vi "log.vi"(8 "error in (no error)":errorcluster, 10 "log_entry":T1 {"datetime" format="%<%x %.3X>T"}, 11 "console.provider in":refnum<class "console.provider.lvclass">) -> (0 "error out":errorcluster, 3 "console.provider out":refnum<class "console.provider.lvclass">)   [LabVIEW 2021, in "console.provider.lvclass"]
uses:
  console.provider.lvclass
  Z:/Projects/DIT/lv-default-repo/source/system.logging.provider/system.logging.provider.lvclass
  system.logging/log_entry.ctl
  system.logging/severity.ctl
  system.logging.provider.lvclass/system.logging.provider.ctl
  console.provider.lvclass/console.provider.ctl
  system.logging.provider.lvclass
  system.logging/system.logging.lvclass
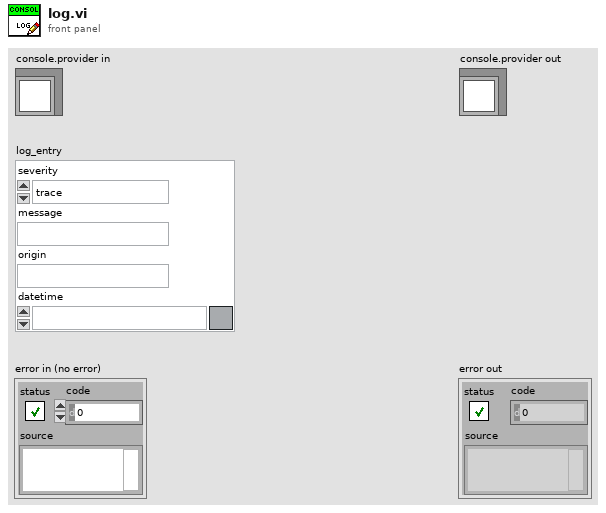
[diagram p1: front panel]
types:
  T1 = typedef "system.logging.lvclass/log_entry.ctl" = cluster{"severity":T2, "message":string, "origin":string, "datetime":timestamp}
  T2 = typedef "system.logging.lvclass/severity.ctl" = enum8{"trace", "debug", "info", "warning", "error"}
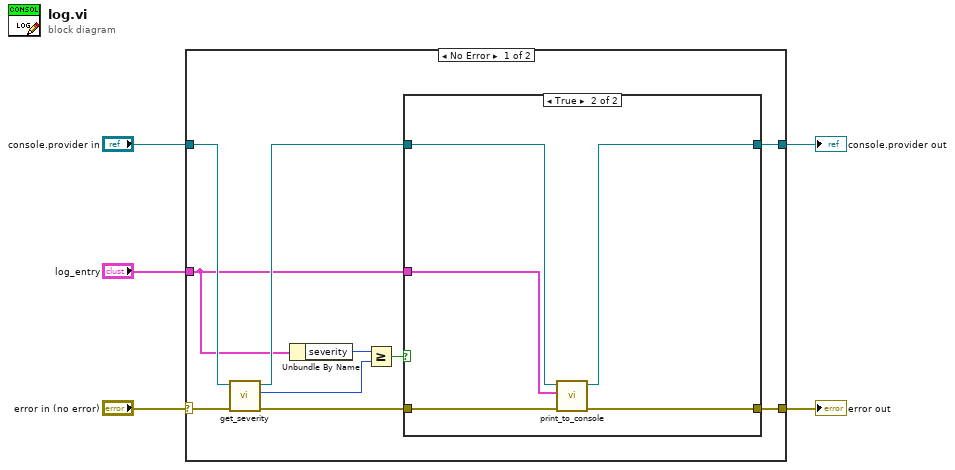
[diagram p0: block diagram]
diagram:
  n1 = case shown="No Error" "error in (no error)" {
    selector: "error in (no error)" -> [w15 w24]
    tunnel: [w8 w24] -> w1
    tunnel: [w7 w23] -> w4
    tunnel: "console.provider in" -> [w14 w23]
    tunnel: "log_entry" -> [w6 _]
    frame No Error {
      n2 = call "get_severity.vi"("error in (no error)"=w15, "system.logging.provider in"=w14) -> ("error out"=w10:errorcluster, "severity"=w12:T2, "system.logging.provider out"=w9:refnum<class "console.provider.lvclass">)  [unwired: 7 in]
      n3 = Unbundle By Name(w6) -> ("severity"=w13:T2)
      n4 = Greater Or Equal?(x=w13, y=w12) -> (x >= y?=w11:bool)
      n5 = case shown="True" w11 {
        tunnel: w10 -> [w17 w22]
        tunnel: w9 -> [w16 w21]
        tunnel: [w17 w18] -> w8
        tunnel: [w16 w20] -> w7
        tunnel: w6 -> [_ w19]
        frame False {
          # "Discard, entry"
        }
        frame True {
          n6 = call "print_to_console.vi"("error in (no error)"=w22, "log"=w19, "console.provider in"=w21) -> ("error out"=w18:errorcluster, "console.provider out"=w20:refnum<class "console.provider.lvclass">)  [unwired: 7 in]
        }
      }
    }
    frame Error {
    }
  }
  "error out" <- w1
  "console.provider out" <- w4
